vi "Write Sub panel prod.vi"(8 "error in (no error)":errorcluster, 10 "Sub panel prod":refnum<vi>, 11 "coffee Actor in":refnum<class "coffee Actor.lvclass">) -> (0 "error out":errorcluster, 3 "coffee Actor out":refnum<class "coffee Actor.lvclass">)   [LabVIEW 2019, in "coffee Actor.lvlib" / "coffee Actor.lvclass"]
uses:
  coffee Actor.lvclass
  coffee Actor.lvclass/coffee Actor.ctl
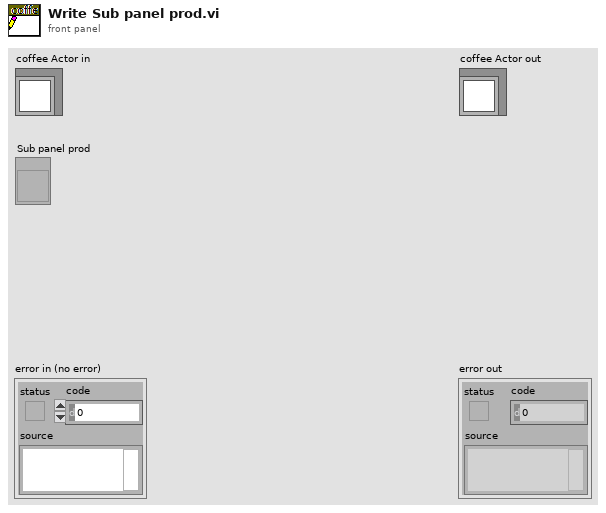
[diagram p1: front panel]
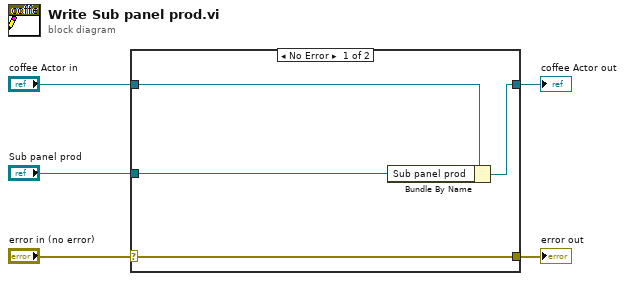
[diagram p0: block diagram]
diagram:
  n1 = case shown="No Error" "error in (no error)" {
    selector: "error in (no error)" -> [w9 w10]
    tunnel: [w9 w10] -> w4
    tunnel: [w7 w11] -> w2
    tunnel: "coffee Actor in" -> [w8 w11]
    tunnel: "Sub panel prod" -> [w6 _]
    frame No Error {
      n2 = Bundle By Name(cluster=w8, "Sub panel prod"=w6) -> (w7:refnum<class "coffee Actor.lvclass">)
    }
    frame Error {
    }
  }
  "error out" <- w4
  "coffee Actor out" <- w2
